vi "Adjust_VI_Properties.vi"(6 "VI refnum in":refnum<vi>, 8 "error in (no error)":errorcluster, 9 "sourceInclusion":T3, 10 "properties in":T1[](array[typedef]), 11 "AB_WebService in":refnum<class "AB_WebService.lvclass">) -> (0 "error out":errorcluster, 1 "defaultSaveLevel":u32, 2 "properties out":T1[](array[typedef]), 3 "AB_WebService out":refnum<class "AB_WebService.lvclass">)   [LabVIEW 2020, in "AB_WebService.lvclass"]
uses:
  <vilib>/AppBuilder/AB_Classes/WebService/AB_WebService.lvclass
  e:/builds/penguin/labview/branches/2020/dev/dist/vi.lib/AppBuilder/AB_Classes/TargetFile/AB_Targetfile.lvclass
  <vilib>/AppBuilder/AB_Source_Inclusion.ctl
  <vilib>/AppBuilder/AB_Source_Properties.ctl
  <vilib>/AppBuilder/AB_Source_Property_Type.ctl
  <vilib>/AppBuilder/AB_Classes/TargetFile/AB_Targetfile.lvclass
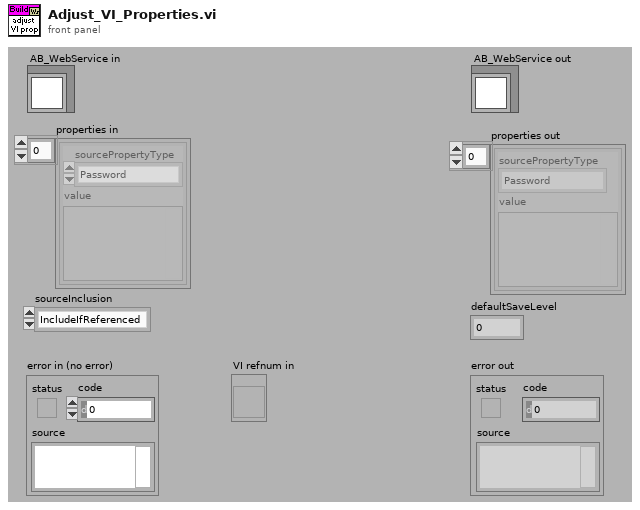
[diagram p1: front panel]
types:
  T1 = typedef "AB_Source_Properties.ctl" = cluster{"sourcePropertyType":T2, "value":variant}
  T2 = typedef "AB_Source_Property_Type.ctl" = enum16{"Remove block diagram", "Remove front panel", "Password", "Window has title bar", "Show menu bar", "Show vertical scroll bar", "Show horizontal scroll bar", "Show toolbar", "Show Abort button", "Show fp when called", "Window behavior", "Allow user to close window", "Window run-time position", "Run when opened", "Allow debugging", "Auto error handling", "Generate guard code", "Use stack variables", "Expression folding", "Integer only", "Inline subVI"}
  T3 = typedef "AB_Source_Inclusion.ctl" = enum16{"IncludeIfReferenced", "Include", "Exclude", "TopLevel"}
  T4 = typedef "AB_Targetfile.ctl" = cluster{"targetfileName":string, "targetfileGUID":string, "enableDebugging":bool, "versionInfo":cluster{"productName":string, "legalCopyright":string, "companyName":string, "internalName":string, "fileDescription":string}, "eng_consolidatedTypeInfo":string, "fastFileFormat":bool, "eng_LEIFBuildData":u32, "versionIndependent":bool}
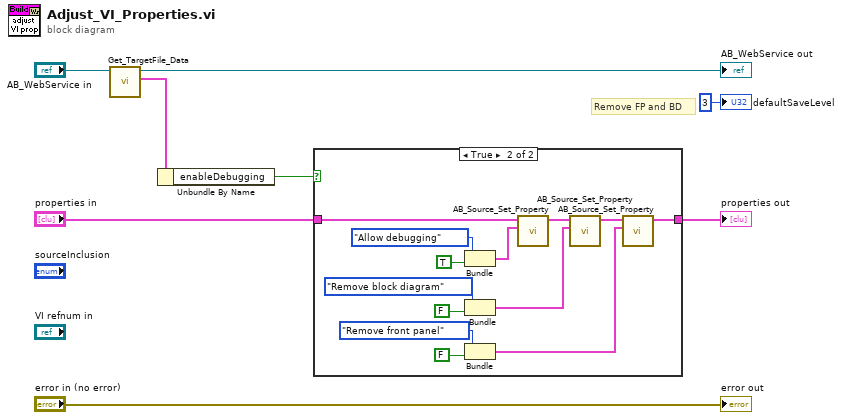
[diagram p0: block diagram]
diagram:
  # "Remove FP and BD"
  n1 = call <vilib>:"Get_TargetFile_Data.vi"("AB_Targetfile in"="AB_WebService in") -> ("data"=w1:T4, "AB_Targetfile out"=→"AB_WebService out":refnum<class "AB_WebService.lvclass">)  [unwired: 8 in, 1 out]
  n2 = Unbundle By Name(w1) -> ("enableDebugging"=w4:bool)
  n3 = case shown="True" w4 {
    tunnel: "properties in" -> [w9 w16]
    tunnel: [w9 w13] -> w5
    frame False {
    }
    frame True {
      n4 = Bundle("sourcePropertyType"=AB_Source_Property_Type."Allow debugging", TRUE) -> (w12:cluster{"sourcePropertyType":T2, bool})  [unwired: 1 out]
      n5 = Bundle("sourcePropertyType"=AB_Source_Property_Type."Remove block diagram", FALSE) -> (w11:cluster{"sourcePropertyType":T2, bool})  [unwired: 1 out]
      n6 = Bundle("sourcePropertyType"=AB_Source_Property_Type."Remove front panel", FALSE) -> (w10:cluster{"sourcePropertyType":T2, bool})  [unwired: 1 out]
      n7 = call <vilib>:"AB_Source_Set_Property.vi"("sourceProperty"=w12, "sourceProperties in"=w16) -> ("sourceProperties out"=w15:T1[])  [unwired: 1 in, 8 out]
      n8 = call <vilib>:"AB_Source_Set_Property.vi"("sourceProperty"=w11, "sourceProperties in"=w15) -> ("sourceProperties out"=w14:T1[])  [unwired: 1 in, 8 out]
      n9 = call <vilib>:"AB_Source_Set_Property.vi"("sourceProperty"=w10, "sourceProperties in"=w14) -> ("sourceProperties out"=w13:T1[])  [unwired: 1 in, 8 out]
    }
  }
  "properties out" <- w5
  "error out" <- "error in (no error)"
  "defaultSaveLevel" <- u32 3 ("defaultSaveLevel")
